vi "Write Controller Enqueuer.vi"(10 "Controller Enqueuer":refnum<class "Message Enqueuer.lvclass">, 11 "Cooler in":refnum<class "Cooler.lvclass">) -> (3 "Cooler out":refnum<class "Cooler.lvclass">)   [LabVIEW 2025, in "Cooler.lvlib" / "Cooler.lvclass"]
doc: "Writes the enqueuer that is used to send messages to the controller. You may pass a Not A Refnum enqueuer as input, indicating that no controller is controlling this cooler."
uses:
  Cooler.lvclass
  <vilib>/ActorFramework/Message Enqueuer/Message Enqueuer.lvclass
  Cooler.lvclass/Cooler.ctl
  <vilib>/ActorFramework/Message Enqueuer/Message Priority.ctl
  Cooler Controller/Update Current Temperature Msg/Update Current Temperature Msg.lvclass/Update Current Temperature Msg.ctl
  <vilib>/ActorFramework/Message Enqueuer/Message Enqueuer.lvclass/Message Enqueuer.ctl
  <vilib>/ActorFramework/Message Enqueuer/Enqueue.vi
  Cooler Controller/Update Current Temperature Msg/Update Current Temperature Msg.lvclass
  C:/Program Files/National Instruments/LabVIEW 2025/vi.lib/ActorFramework/Message/Message.lvclass
  <vilib>/ActorFramework/Message Priority Queue/Priority Enqueue.vi
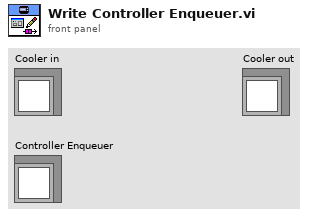
[diagram p1: front panel]
types:
  T1 = typedef "Actor Framework.lvlib/Message Enqueuer.lvclass/Message Priority.ctl" = enum16{"Low", "Normal", "High"}
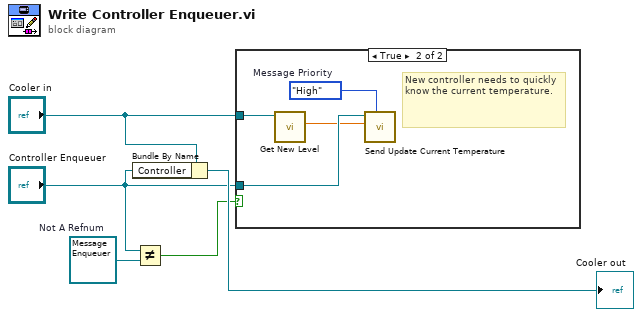
[diagram p0: block diagram]
diagram:
  w4 = refnum<class "Message Enqueuer.lvclass"> refnum  # Not A Refnum
  n1 = Bundle By Name(cluster="Cooler in", "Controller"="Controller Enqueuer") -> (→"Cooler out":refnum<class "Cooler.lvclass">)
  n2 = Not Equal?(x="Controller Enqueuer", y=w4) -> (x != y?=w3:bool)
  n3 = case shown="True" w3 {
    tunnel: "Controller Enqueuer" -> [_ w9]
    tunnel: "Cooler in" -> [_ w7]
    frame False {
    }
    frame True {
      w6 = Message_Priority."High"  # Message Priority
      # "New controller needs to quickly know the current temperature."
      n4 = call-dynamic "Get New Level.vi"("Cooler in"=w7) -> ("Level"=w8:dbl)  [unwired: 8 in, 2 out]
      n5 = call "Send Update Current Temperature.vi"("Message Priority (Normal)"=w6, "Current Temperature"=w8, "Message Enqueuer"=w9) -> ()  [unwired: 8 in, 1 out]
    }
  }
